vi "_XNET Create Session.vi"(0 "database (empty)":string, 1 "interface":refnum<k21>, 2 "mode":u32, 5 "cluster (empty)":string, 7 "signal/frame list (empty)":string[](array[string]), 11 "error in (no error)":errorcluster) -> (4 "session out":refnum<k21>, 15 "error out":errorcluster)   [LabVIEW 2018]
doc: "Internal subVI of NI-XNET.\n\nThis is the actual implementation of the Create Session call to the NI-XNET library. Higher level VIs convert specific LabVIEW I/O name classes into strings, then call this subVI."
uses:
  nixlvapi.dll
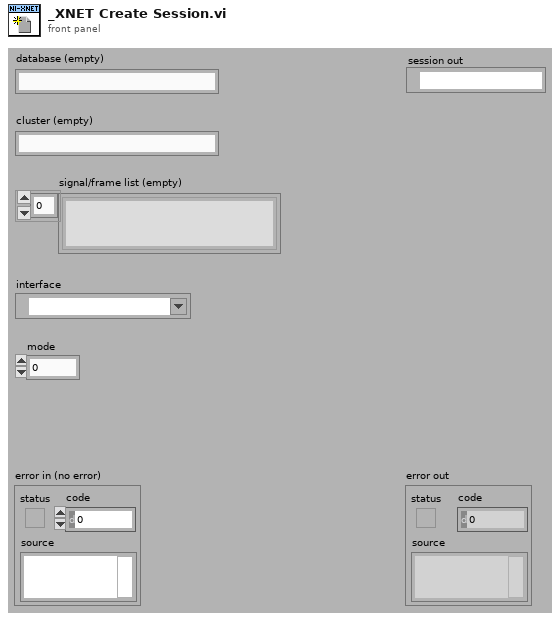
[diagram p1: front panel]
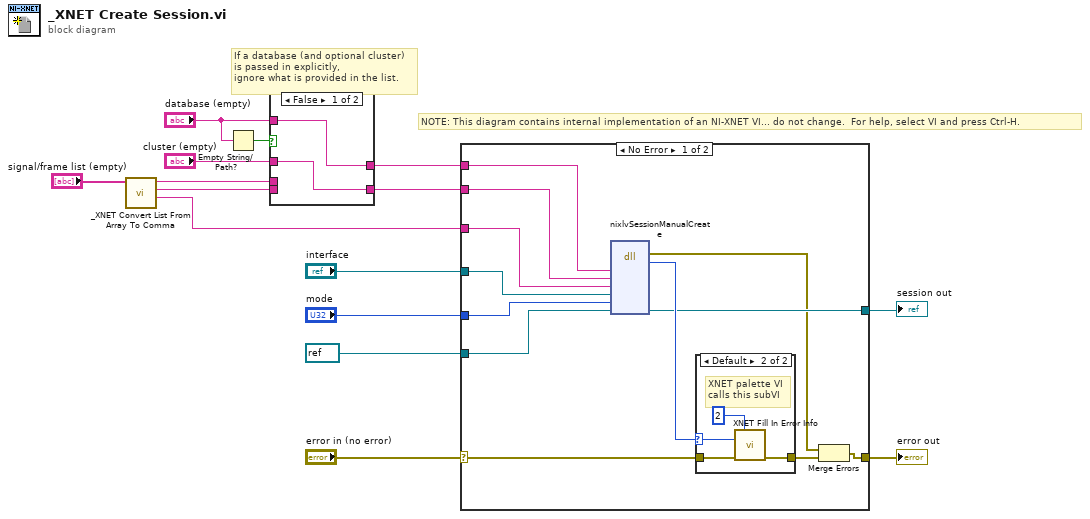
[diagram p0: block diagram]
diagram:
  # "If a database (and optional cluster)\nis passed in explicitly,\nignore what is provided in the list."
  # "NOTE: This diagram contains internal implementation of an NI-XNET VI... do not change.  For help, select VI and press Ctrl-H."
  n1 = call "_XNET Convert List From Array To Comma.vi"("list in"="signal/frame list (empty)") -> ("commaSeparatedList out"=w4:string, "cluster out"=w5:string, "database out"=w6:string)  [unwired: 1 in, 6 out]
  n2 = Empty String/Path?(string/path="database (empty)") -> (empty?=w9:bool)
  n3 = case shown="False" w9 {
    tunnel: "database (empty)" -> [w17 _]
    tunnel: "cluster (empty)" -> [w16 _]
    tunnel: w6 -> [_ w19]
    tunnel: w5 -> [_ w18]
    tunnel: [w17 w19] -> w3
    tunnel: [w16 w18] -> w2
    frame False {
    }
    frame True {
    }
  }
  n4 = case shown="No Error" "error in (no error)" {
    selector: "error in (no error)" -> [w31 w38]
    tunnel: [w21 w38] -> w15
    tunnel: [w22 refnum<k21> refnum ("taskRefObjectPtr")] -> w13
    tunnel: "interface" -> [w28 _]
    tunnel: "mode" -> [w29 _]
    tunnel: w4 -> [w27 _]
    tunnel: w3 -> [w25 _]
    tunnel: w2 -> [w26 _]
    tunnel: refnum<k21> refnum ("session out") -> [w23 _]
    frame No Error {
      n5 = dll-call lib="nixlvapi.*" fn="nixlvSessionManualCreate"("database"=w25, "cluster"=w26, "commaSeparatedList"=w27, "interfaceName"=w28, "mode"=w29, "refObjPtr"=w23) -> (error out=w20:errorcluster, "return type"=w30:i32, "refObjPtr"=w22:refnum<k21>)  [unwired: 7 in, 2 out]
      n6 = case shown="Default" w30 {
        selector: w30 -> [_ w34]
        tunnel: w31 -> [w32 w35]
        tunnel: [w32 w36] -> w24
        frame 0 {
        }
        frame Default {
          # "XNET palette VI\ncalls this subVI"
          n7 = call "XNET Fill In Error Info.vi"("depth (1)"=2 ("depth"), "status code"=w34, "error in"=w35) -> ("error out"=w36:errorcluster)  [unwired: 12 out]
        }
      }
      n8 = Merge Errors(w20, w24) -> (w21:errorcluster)
    }
    frame Error {
    }
  }
  "error out" <- w15
  "session out" <- w13
